vi "PID_REG.vi"(0 "History Data 2":dbl[](array[numeric]), 1 "milliseconds to wait":u32, 2 "History Data in":dbl[](array[numeric]), 5 "Coerce?":bool, 7 "Tout":dbl, 9 "Default værdier":T3, 12 "SP":dbl, 13 "element":T4, 14 "PID?":bool) -> (4 "Cluster":T2, 6 "History Data":dbl[](array[numeric]), 8 "Tout out":dbl, 15 "P I D":T1)   [LabVIEW 2022 SP3]
uses:
  TypeDefs/P_I_D_Data_type.ctl
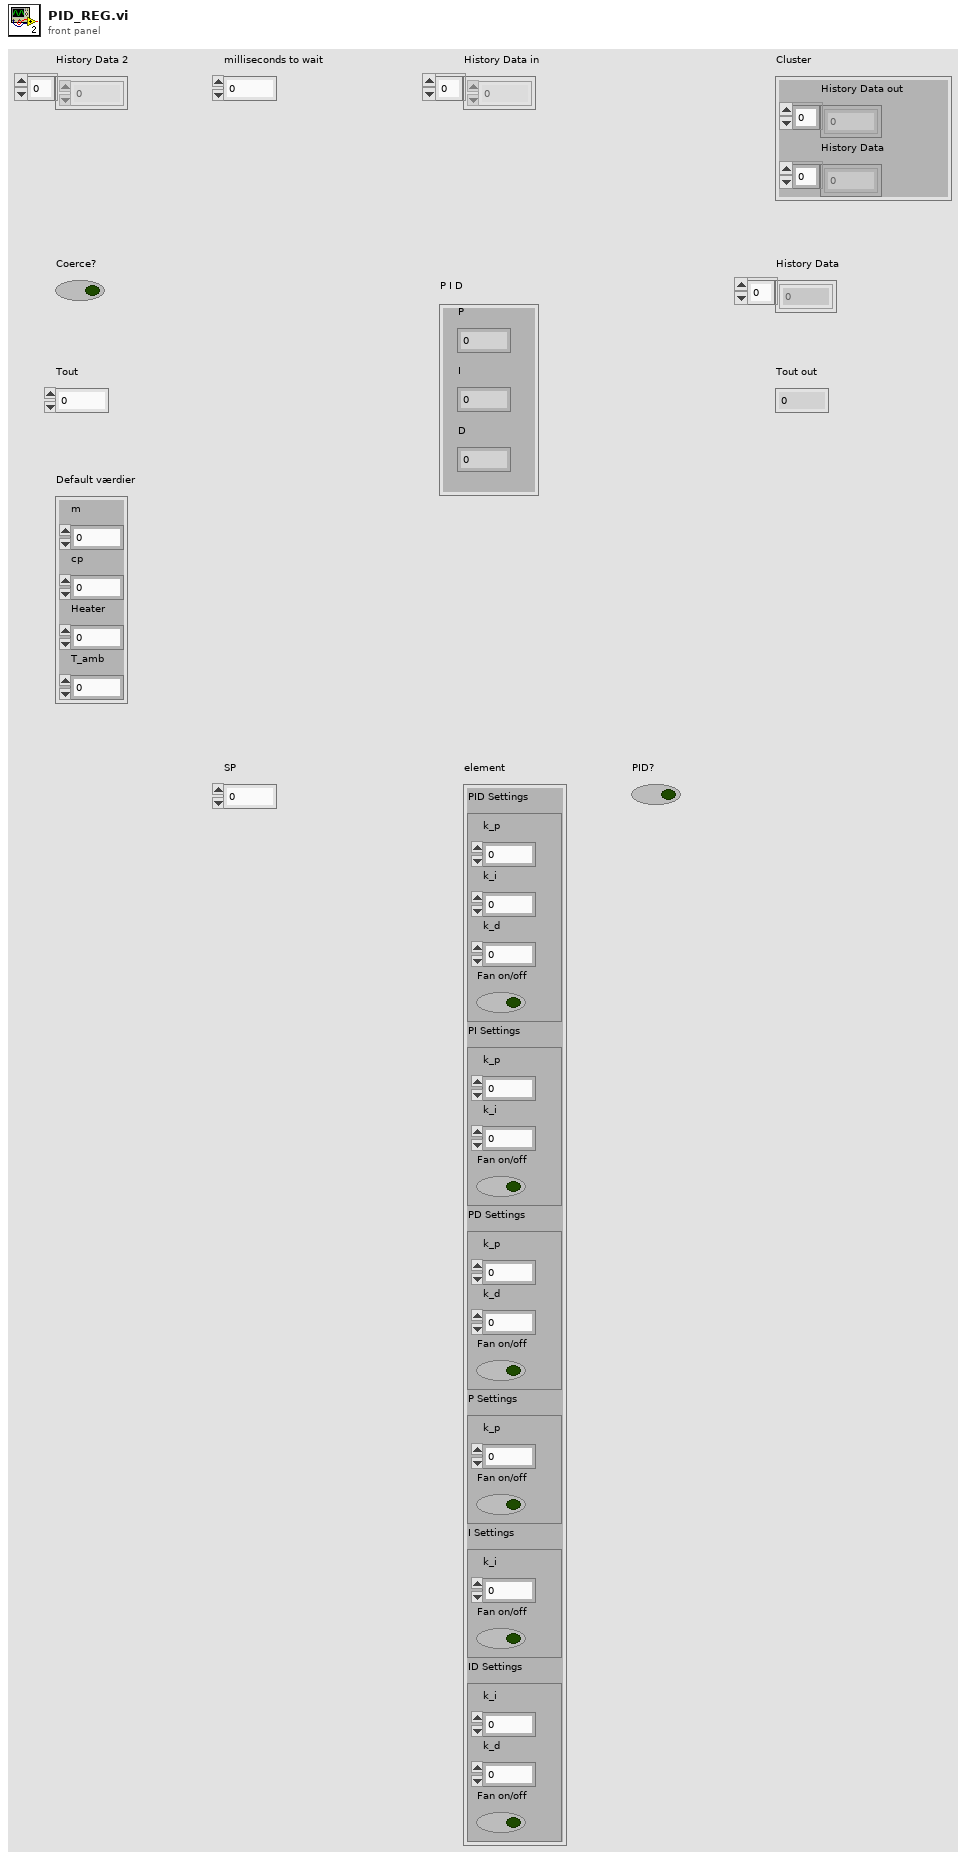
[diagram p1: front panel]
types:
  T1 = typedef "P_I_D_Data_type.ctl" = cluster{"P":dbl, "I":dbl, "D":dbl}
  T2 = cluster{"History Data out":dbl[], "History Data":dbl[]}
  T3 = cluster{"m":dbl, "cp":dbl, "Heater":dbl, "T_amb":dbl}
  T4 = cluster{"PID Settings":cluster{"k_p":dbl, "k_i":dbl, "k_d":dbl, "Fan on/off":bool}, "PI Settings":cluster{"k_p":dbl, "k_i":dbl, "Fan on/off":bool}, "PD Settings":cluster{"k_p":dbl, "k_d":dbl, "Fan on/off":bool}, "P Settings":cluster{"k_p":dbl, "Fan on/off":bool}, "I Settings":cluster{"k_i":dbl, "Fan on/off":bool}, "ID Settings":cluster{"k_i":dbl, "k_d":dbl, "Fan on/off":bool}}
  T5 = enum16{"I_REG", "ID_REG", "P_REG", "PI_REG", "PD_REG", "PID_REG"}
  T6 = cluster{"k_p":dbl, "k_i":dbl, "k_d":dbl, "Fan on/off":bool}
  T7 = cluster{"History Data in":dbl[], "History Data 2":dbl[]}
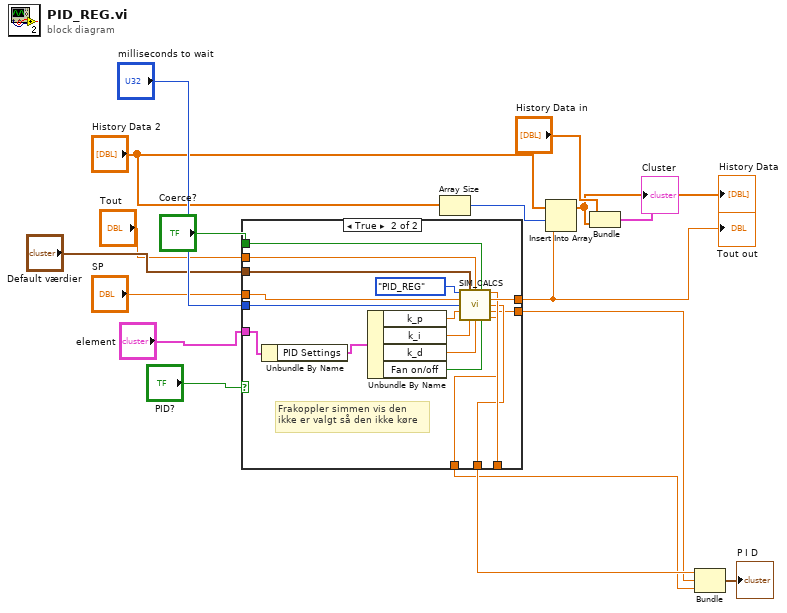
[diagram p0: block diagram]
diagram:
  n1 = case shown="True" "PID?" {
    tunnel: "Tout" -> [_ w31]
    tunnel: "Default værdier" -> [_ w30]
    tunnel: [_ w28] -> w8
    tunnel: "milliseconds to wait" -> [_ w26]
    tunnel: "Coerce?" -> [_ w25]
    tunnel: "SP" -> [_ w24]
    tunnel: "element" -> [_ w23]
    tunnel: [_ w21] -> _
    tunnel: [_ w20] -> w4
    tunnel: [_ w19] -> w3
    tunnel: [_ w18] -> w2
    frame False {
    }
    frame True {
      # "Frakoppler simmen vis den\nikke er valgt så den ikke køre"
      n2 = Unbundle By Name(w23) -> ("PID Settings"=w22:T6)
      n3 = Unbundle By Name(w22) -> ("k_p"=w34:dbl, "k_i"=w33:dbl, "k_d"=w32:dbl, "Fan on/off"=w29:bool)
      n4 = call "SIM_CALCS.vi"("Regulation type"=T5."PID_REG", "Default værdier"=w30, "Tout in"=w31, "Coerce?"=w25, "SP"=w24, "milliseconds to wait"=w26, "k_p"=w34, "k_i"=w33, "k_d"=w32, "Fan on/off"=w29) -> ("u"=w21:dbl, "Tout out"=w28:dbl, "P"=w20:dbl, "I"=w19:dbl, "D"=w18:dbl)  [unwired: 1 in]
    }
  }
  "Tout out" <- w8
  n5 = Array Size(array="History Data 2") -> (size(s)=w7:i32)
  n6 = Insert Into Array(array="History Data 2", index=w7, new element=w8) -> (w10:dbl[])
  "History Data" <- w10
  n7 = Bundle("History Data in"="History Data in", "History Data 2"=w10) -> (→"Cluster":T7)  [unwired: 1 in]
  n8 = Bundle("P"=w4, "I"=w3, "D"=w2) -> (→"P I D":cluster{"P":dbl, "I":dbl, "D":dbl})  [unwired: 1 in]
